vi "QCP_Get_STR.vi"(0 "QCP Data Block In":T1, 1 "QCP Name":string, 3 "Error In":errorcluster) -> (7 "QCP Data Block Out":T1, 8 "Value Out":string, 10 "Error Out":errorcluster)   [LabVIEW 2016]
uses:
  <userlib>/836-Libraries/System/QCP_Support_Code/QCP_Data_Block.ctl
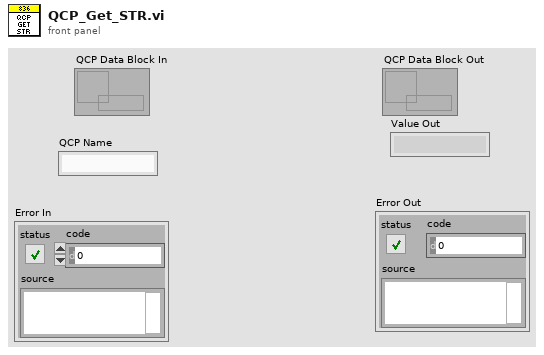
[diagram p1: front panel]
types:
  T1 = typedef "QCP_Data_Block.ctl" = refnum<data-value>
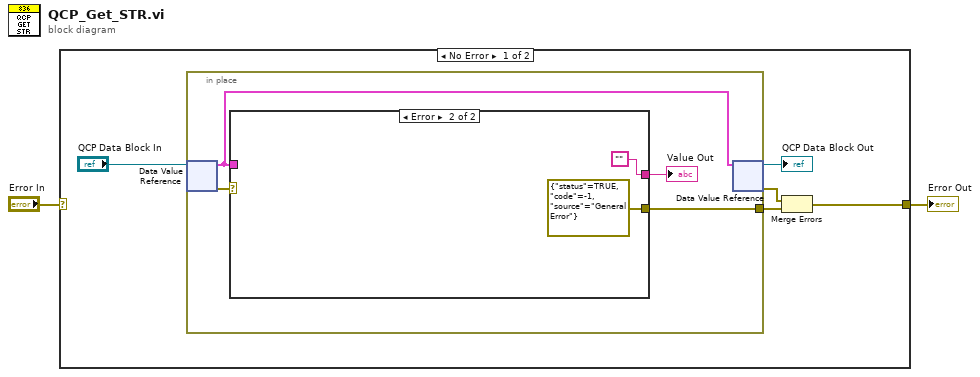
[diagram p0: block diagram]
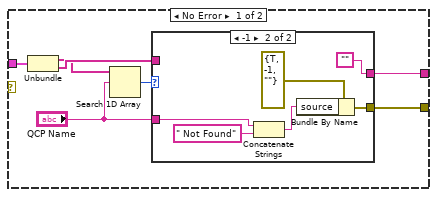
[diagram p2: hidden frame]
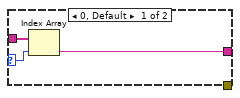
[diagram p3: hidden frame]
diagram:
  n1 = case shown="No Error" "Error In" {
    selector: "Error In" -> [_ w30]
    tunnel: [w3 w30] -> w1
    frame No Error {
      n2 = in-place {
        in-place-border: [w8] -> w5
        n3 = in-place-dvr #1("QCP Data Block In") -> (w10:cluster{string[], string[]}, w11:errorcluster)
        n4 = case shown="Error" w11 {
          tunnel: w10 -> [w15 _]
          tunnel: [w14 ""] -> w9
          tunnel: [w12 errorcluster {"status"=TRUE, "code"=-1, "source"="General Error"} ("error constant")] -> w8
          frame No Error {
            n5 = Unbundle(w15) -> (w17:string[], w18:string[])
            n6 = Search 1D Array(1D array=w17, element="QCP Name") -> (index of element=w16:i32)  [unwired: 1 out]
            n7 = case shown="-1" w16 {
              selector: w16 -> [w21 _]
              tunnel: [w19 ""] -> w14
              tunnel: w18 -> [w20 _]
              tunnel: "QCP Name" -> [_ w23]
              tunnel: [_ w22] -> w12
              frame 0, Default {
                n8 = Index Array(array=w20, index=w21) -> (element=w19:string)
              }
              frame -1 {
                n9 = Concatenate Strings(w23, " Not Found") -> (w24:string)
                n10 = Bundle By Name(cluster=errorcluster {"status"=TRUE, "code"=-1, "source"=""} ("error constant"), "source"=w24) -> (w22:errorcluster)
              }
            }
          }
          frame Error {
          }
        }
        "Value Out" <- w9
        n11 = in-place-dvr #1(w10) -> (→"QCP Data Block Out":T1, w4:errorcluster)
      }
      n12 = Merge Errors(w4, w5) -> (w3:errorcluster)
    }
    frame Error {
    }
  }
  "Error Out" <- w1
